vi "object selector (SubVI).vi"(10 "output array":string[][](array[string]), 11 "Numeric":i32) -> (2 "Cluster":cluster{"Object":i32, i32}, 3 "Cluster 2":cluster{i32, "Object":i32})   [LabVIEW 2020]
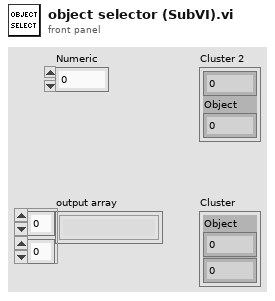
[diagram p1: front panel]
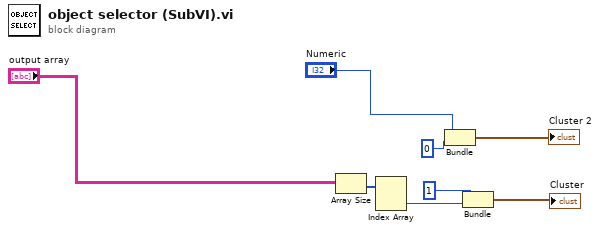
[diagram p0: block diagram]
diagram:
  n1 = Array Size(array="output array") -> (size(s)=w7:i32[])
  n2 = Index Array(array=w7) -> (element #2=w8:i32)  [unwired: 2 in, 1 out]
  n3 = Bundle("Numeric"="Numeric", "Object"=0) -> (→"Cluster 2":cluster{"Numeric":i32, "Object":i32})  [unwired: 1 in]
  n4 = Bundle("Object"=1, w8) -> (→"Cluster":cluster{"Object":i32, i32})  [unwired: 1 in]
